vi "Unique Array.vi"(10 "Sort? (T)":bool=TRUE, 11 "Array":string[](array[string])) -> (3 "Unique Array":string[](array[string]))   [LabVIEW 2019, in "LSS.lvlib"]
doc: "Find unique elements in an array, removing duplicates.\n\n<b>Inputs:</b>\n<b>Array</b> - Array with duplicates.\n\n<b>Outputs:</b>\n<b>Unique Array</b> - Array with duplicates removed."
uses:
  LSS.lvlib
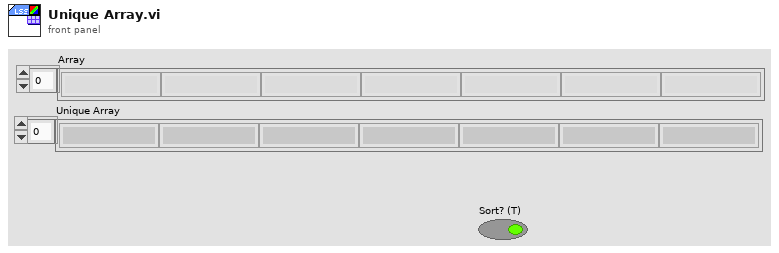
[diagram p1: front panel]
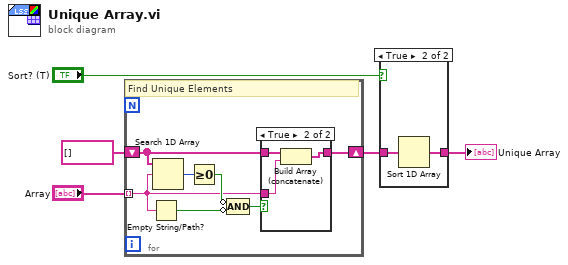
[diagram p0: block diagram]
diagram:
  n1 = for {
    shift-right: [w10] -> w3
    shift-left: string[] [] ("Array") -> [w9]
    tunnel: "Array" -> [w8] mode=indexing
    # "Find Unique Elements"
    n2 = Empty String/Path?(string/path=w8) -> (empty?=w6:bool)
    n3 = Search 1D Array(1D array=w9, element=w8) -> (index of element=w12:i32)  [unwired: 1 in]
    n4 = Greater Or Equal To 0?(x=w12) -> (x >= 0?=w11:bool)
    n5 = Compound Arithmetic op=AND(invert w11, invert w6) -> (w7:bool)
    n6 = case shown="True" w7 {
      tunnel: [w13 w14] -> w10
      tunnel: w9 -> [w13 w16]
      tunnel: w8 -> [_ w15]
      frame False {
      }
      frame True {
        n7 = Build Array (concatenate)(w16, w15) -> (w14:string[])
      }
    }
  }
  n8 = case shown="True" "Sort? (T)" {
    tunnel: w3 -> [w17 w19]
    tunnel: [w17 w18] -> w2
    frame False {
    }
    frame True {
      n9 = Sort 1D Array(array=w19) -> (sorted array=w18:string[])
    }
  }
  "Unique Array" <- w2
